vi "Phase Measure.vi"() -> ()   [LabVIEW 2009]
uses:
  <vilib>/DAQmx/configure/timing.llb/DAQmx Timing (Sample Clock).vi
  <vilib>/DAQmx/configure/trigger.llb/DAQmx Start Trigger (Digital Edge).vi
  <vilib>/DAQmx/create/channels.llb/DAQmx Create Channel (AI-Voltage-Basic).vi
  <vilib>/Utility/error.llb/DialogType.ctl
  <vilib>/DAQmx/read.llb/DAQmx Read (Analog Wfm 1Chan NSamp).vi
panel:
  out "Acquisition Sequence":waveform(dbl)(graph)
  in  "stop":bool
  in  "Maximum Value 2":dbl=10.0 caption="Maximum Value" format="%0.2f"
  in  "Minimum Value 2":dbl=-10.0 caption="Minimum Value" format="%0.2f"
  in  "Sample Rate":dbl=10000.0 caption="Sample Rate (Hz)" format="%0.2f"
  in  "Physical Channel 2":tag="Dev1/ai0" caption="Physical Channel"
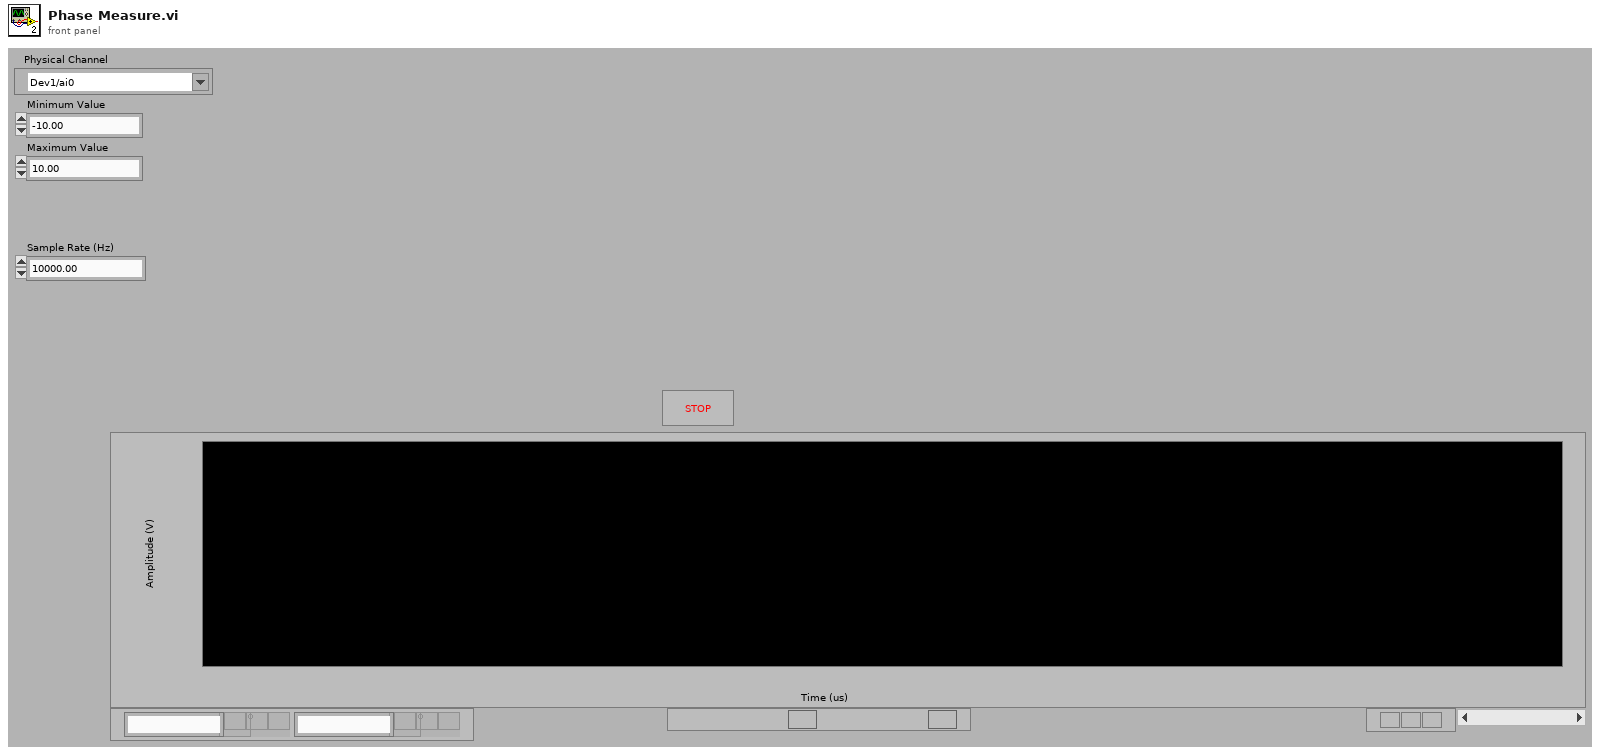
[diagram p1: front panel]
types:
  T1 = typedef "DialogType.ctl" = u16
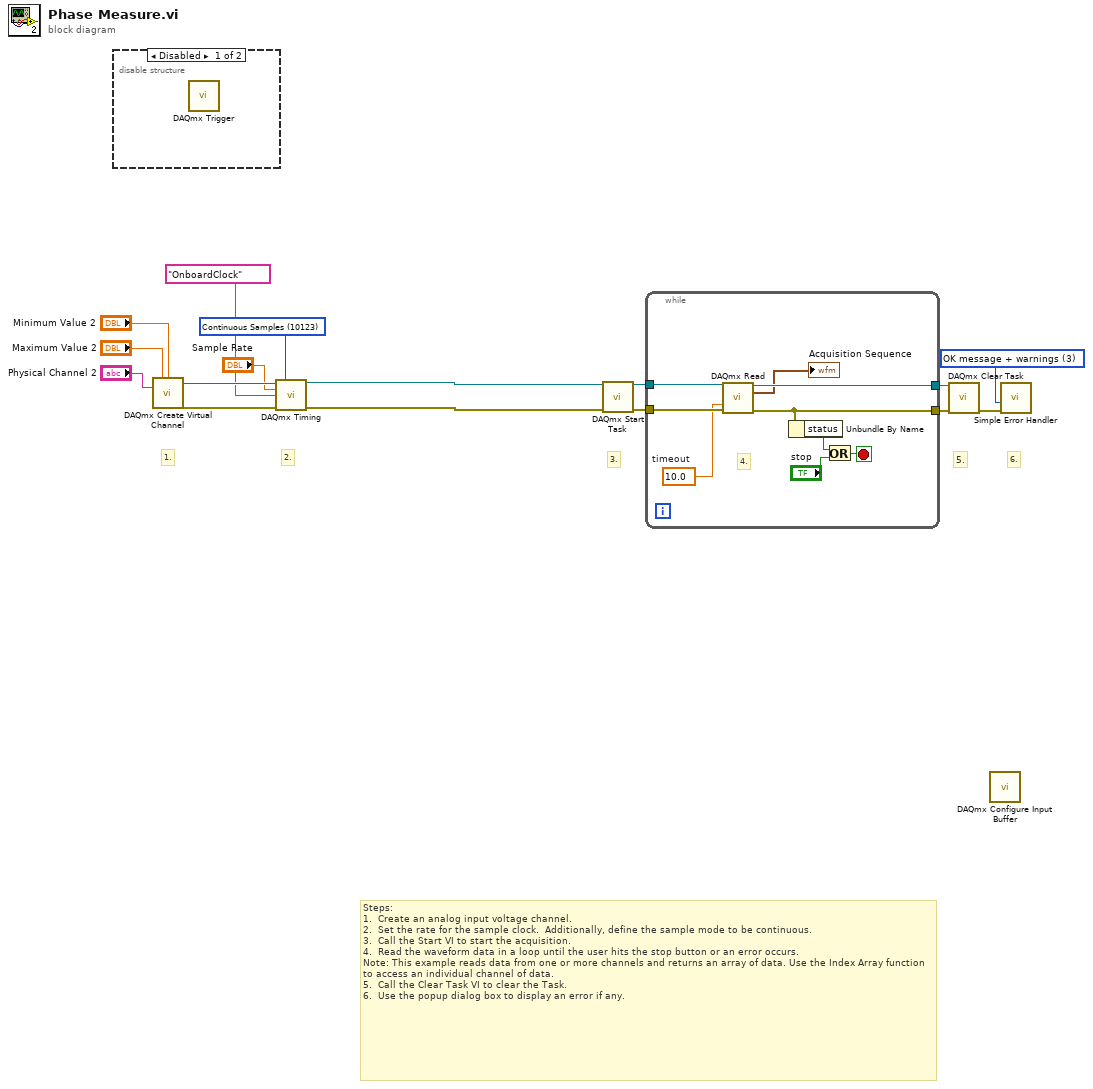
[diagram p0: block diagram]
diagram:
  w2 = T1 3 items=["no dialog", "OK message", "continue or stop message", "OK message + warnings", "continue/stop + warnings"] ("type of dialog (OK msg:1)")
  w7 = 10123 items=["Finite Samples"=10178, "Continuous Samples"=10123] ("sample mode")
  # "6."
  # "5."
  # "Steps: \n1.  Create an analog input voltage channel.\n2.  Set the rate for the sample clock.  Additionally, define the sample mode to be continuous.\n3.  Call the Start VI to start the acquisition.\n4.  Read the waveform data in a loop until the user hits the stop button or an error occurs.\nNote: This example reads data from one or more channels and returns an array of data. Use the Index Array function to access an individual channel of data.\n5.  Call the Clear Task VI to clear the Task.\n6.  Use the popup dialog box to display an error if any."
  # "3."
  # "2."
  # "1."
  n1 = disable-structure shown="Disabled" {
    frame #0 {
      n2 = call-poly <vilib>:"DAQmx Trigger.vi"() -> ()  [unwired: 5 in, 11 out]
    }
    frame #1 {
    }
  }
  n3 = call-poly <vilib>:"DAQmx Create Virtual Channel.vi"("maximum value"="Maximum Value 2", "minimum value"="Minimum Value 2", "physical channels"="Physical Channel 2") -> ("task out"=w11:refnum<k21>, "error out"=w14:errorcluster)  [unwired: 6 in, 5 out]
  n4 = call-poly <vilib>:"DAQmx Timing.vi"("task/channels in"=w11, "sample mode"=w7, "rate"="Sample Rate", "source"=tag "OnboardClock", "error in"=w14) -> ("task out"=w6:refnum<k21>, "error out"=w5:errorcluster)  [unwired: 2 in, 7 out]
  n5 = call <vilib>:"DAQmx Start Task.vi"("task/channels in"=w6, "error in"=w5) -> ("task out"=w10:refnum<k21>, "error out"=w13:errorcluster)  [unwired: 12 out]
  n6 = while {
    tunnel: w13 -> [w25]
    tunnel: w10 -> [w24]
    tunnel: [w23] -> w9
    tunnel: [w22] -> w4
    stop <- w20 stop-if-true
    w18 = 10.0  # timeout
    # "4."
    n7 = call-poly <vilib>:"DAQmx Read.vi"("task/channels in"=w24, "timeout"=w18, "error in"=w25) -> ("task out"=w23:refnum<k21>, "data"=→"Acquisition Sequence":waveform(dbl), "error out"=w22:errorcluster)  [unwired: 1 in, 9 out]
    n8 = Unbundle By Name(w22) -> ("status"=w21:bool)
    n9 = Or(x=w21, y="stop") -> (x .or. y?=w20:bool)
  }
  n10 = call <vilib>:"DAQmx Clear Task.vi"("task in"=w9, "error in"=w4) -> ("error out"=w12:errorcluster)  [unwired: 13 out]
  n11 = call <vilib>:"DAQmx Configure Input Buffer.vi"() -> ()  [unwired: 14 in, 2 out]
  n12 = call <vilib>:"Simple Error Handler.vi"("type of dialog (OK msg:1)"=w2, "error in (no error)"=w12) -> ()  [unwired: 8 out]
